vi "spot_gen_tester.vi"() -> ()   [LabVIEW 2021]
panel:
  in  "PW":u16=100
  in  "Rx_detect_param":T1={"detection bar"=2500.0, "max gap"=2, "max PW"=500, "min PW"=10}
  out "Array":cluster{u16, u16, u32}[](array[cluster])
  out "size(s)":i32
  in  "num_of loops":i32=60000
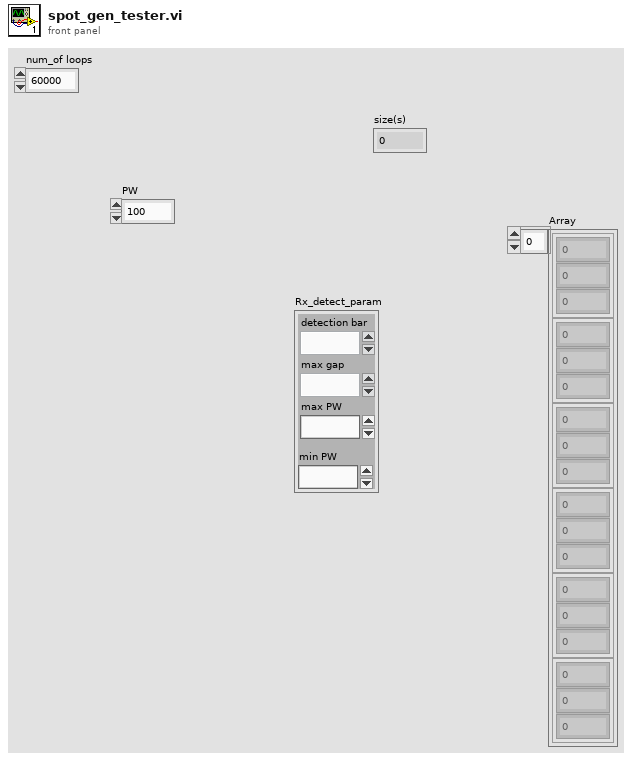
[diagram p1: front panel]
types:
  T1 = cluster{"detection bar":fxp<+,64,63>, "max gap":u8, "max PW":u16, "min PW":u16}
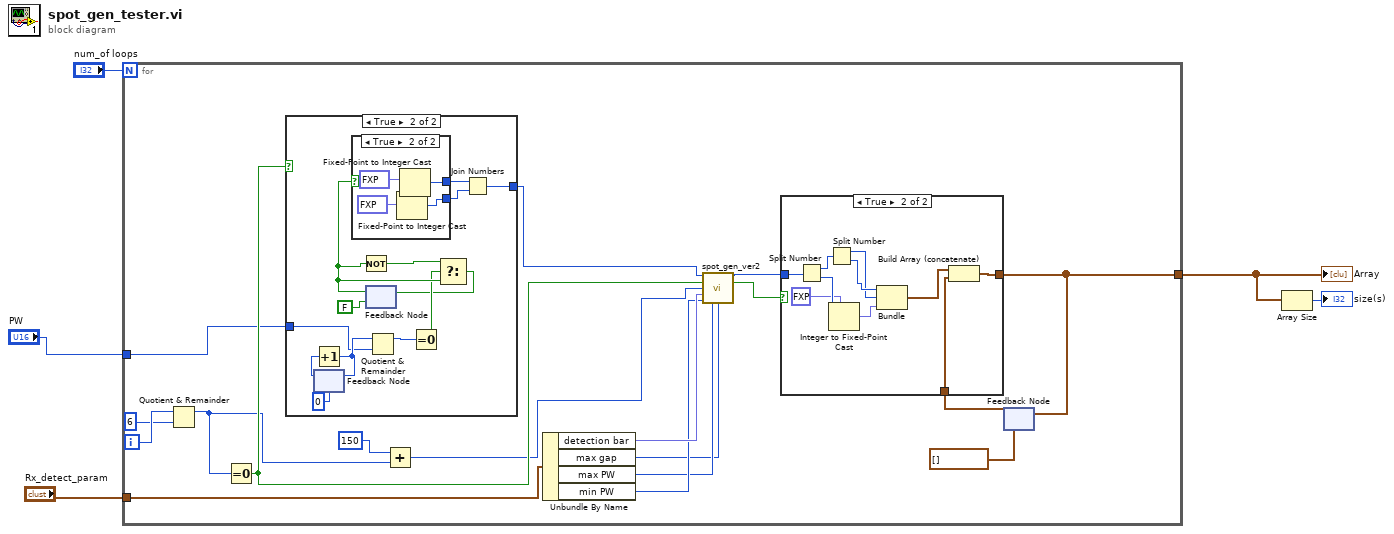
[diagram p0: block diagram]
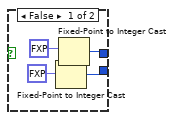
[diagram p3: hidden frame]
diagram:
  n1 = for {
    N: "num_of loops" -> [_]
    tunnel: [w22] -> w4
    tunnel: "Rx_detect_param" -> [w19]
    tunnel: "PW" -> [w10]
    i -> [w21]
    n2 = Quotient & Remainder(x=w21, y=6) -> (x-y*floor(x/y)=w7:i32)  [unwired: 1 out]
    n3 = Equal To 0?(x=w7) -> (x = 0?=w12:bool)
    n4 = case shown="True" w12 {
      tunnel: [_ w25] -> w11
      tunnel: w10 -> [_ w24]
      frame False {
      }
      frame True {
        n5 = feedback #1(u16 0 ("data index 2")) -> (w35:u16)
        n6 = Increment(x=w35) -> (x+1=w32:u16)
        n7 = feedback-in #1(w32) -> ()
        n8 = feedback #2(FALSE) -> (w31:bool)
        n9 = case shown="True" w31 {
          tunnel: [w38 w44] -> w27
          tunnel: [w37 w43] -> w26
          frame False {
            n10 = Fixed-Point to Integer Cast(1:fxp<+/-,32,31> 7.0 ("fixed-point")) -> (0:w37:i32)
            n11 = Fixed-Point to Integer Cast(1:fxp<+/-,32,31> 15.0 ("fixed-point")) -> (0:w38:i32)
          }
          frame True {
            n12 = Fixed-Point to Integer Cast(1:fxp<+/-,32,31> 4500.0 ("fixed-point")) -> (0:w43:i32)
            n13 = Fixed-Point to Integer Cast(1:fxp<+/-,32,31> 4500.0 ("fixed-point")) -> (0:w44:i32)
          }
        }
        n14 = Not(x=w31) -> (.not. x?=w30:bool)
        n15 = Quotient & Remainder(x=w32, y=w24) -> (x-y*floor(x/y)=w33:u16)  [unwired: 1 out]
        n16 = Equal To 0?(x=w33) -> (x = 0?=w29:bool)
        n17 = Select(t=w30, s=w29, f=w31) -> (s? t:f=w28:bool)
        n18 = feedback-in #2(w28) -> ()
        n19 = Join Numbers(hi=w27, lo=w26) -> ((hi.lo)=w25:u64)
      }
    }
    n20 = Add(x=u16 150 ("data index 2"), y=w7) -> (x+y=w6:i32)
    n21 = Unbundle By Name(w19) -> ("detection bar"=w16:fxp<+,64,63>, "max gap"=w13:u8, "max PW"=w14:u16, "min PW"=w15:u16)
    n22 = call "spot_gen_ver2.vi"("FFT_output"=w11, "input valid"=w12, "data index 2"=w6, "amplitude bar"=w16, "min PW"=w15, "max PW 2"=w14, "max gap"=w13) -> ("PDW"=w18:u64, "output valid"=w17:bool)  [unwired: 6 in, 1 out]
    n23 = feedback #3(cluster{u16, u16, "magnitude":fxp<+,32,31>}[] []) -> (w23:cluster{u16, u16, "magnitude":fxp<+,32,31>}[])
    n24 = case shown="True" w17 {
      tunnel: w18 -> [_ w53]
      tunnel: [w45 w55] -> w22
      tunnel: w23 -> [w45 w54]
      frame False {
      }
      frame True {
        n25 = Split Number(x=w53) -> (hi(x)=w52:u32, lo(x)=w48:u32)
        n26 = Split Number(x=w52) -> (hi(x)=w49:u16, lo(x)=w50:u16)
        n27 = Integer to Fixed-Point Cast(fixed-point type=fxp<+,32,31> 0.0 ("magnitude"), integer=w48) -> (fixed-point=w47:fxp<+,32,31>)
        n28 = Bundle(w50, w49, "magnitude"=w47) -> (w51:cluster{u16, u16, "magnitude":fxp<+,32,31>})  [unwired: 1 in]
        n29 = Build Array (concatenate)(w51, w54) -> (w55:cluster{u16, u16, "magnitude":fxp<+,32,31>}[])
      }
    }
    n30 = feedback-in #3(w22) -> ()
  }
  "Array" <- w4
  n31 = Array Size(array=w4) -> (size(s)=→"size(s)":i32)
